vi "airplain.vi"(1 "steering":T1={"control"={"rudder"=-6, "aileron"=-15}, "rotate"={"pitch"=-22, "roll"=-18, "yaw"=158}, "pos"={"x"=0, "y"=0, "z"=-57}} {"control"."rudder" scale=-30.0..30.0; "control"."aileron" scale=-30.0..30.0; "rotate"."pitch" scale=-180.0..180.0; "rotate"."roll" scale=-180.0..180.0; "rotate"."yaw" scale=-180.0..180.0; "pos"."x" scale=-10.0..10.0; "pos"."y" scale=-20.0..20.0; "pos"."z" scale=-200.0..200.0}, 2 "center":cluster{"x":u32, "y":u32}={"x"=65, "y"=58}) -> (0 "picture out 2":picture)   [LabVIEW 2011]
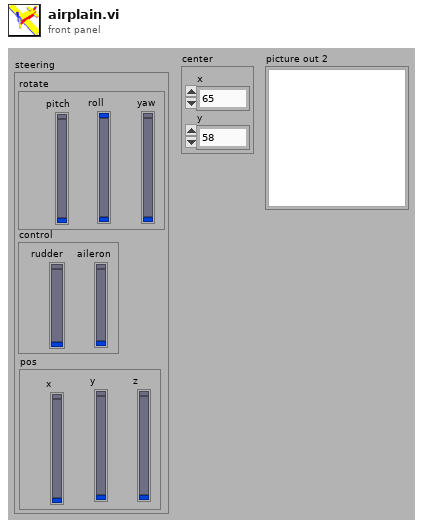
[diagram p1: front panel]
types:
  T1 = cluster{"control":cluster{"rudder":i32, "aileron":i32}, "rotate":cluster{"pitch":i32, "roll":i32, "yaw":i32}, "pos":cluster{"x":i32, "y":i32, "z":i32}}
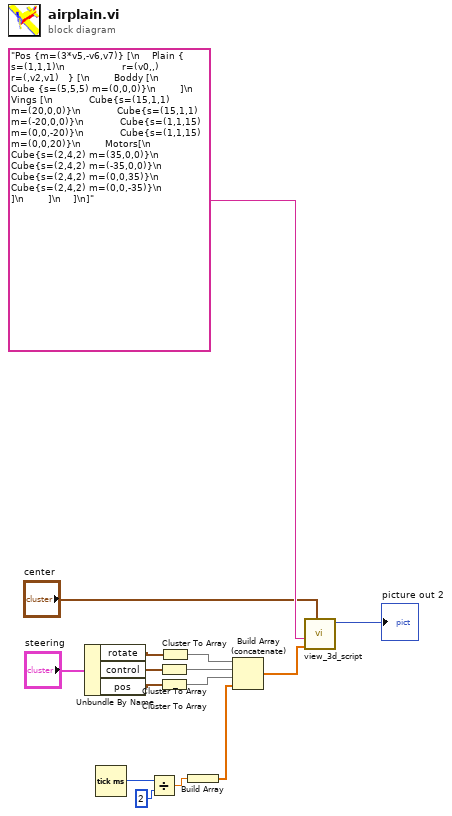
[diagram p0: block diagram]
diagram:
  n1 = Unbundle By Name("steering") -> ("rotate"=w1:cluster{"pitch":i32, "roll":i32, "yaw":i32}, "control"=w2:cluster{"rudder":i32, "aileron":i32}, "pos"=w3:cluster{"x":i32, "y":i32, "z":i32})
  n2 = Tick Count (ms)() -> (millisecond timer value=w10:u32)
  n3 = Divide(x=w10, y=u16 2) -> (x/y=w9:dbl)
  n4 = Cluster To Array(cluster=w2) -> (array=w14:i32[])
  n5 = Cluster To Array(cluster=w3) -> (array=w13:i32[])
  n6 = Cluster To Array(cluster=w1) -> (array=w15:i32[])
  n7 = Build Array(w9) -> (w12:dbl[])
  n8 = Build Array (concatenate)(w15, w14, w13, w12) -> (w8:dbl[])
  n9 = call "view_3d_script.vi"("center"="center", "variables"=w8, "script"="Pos {m=(3*v5,-v6,v7)} [\n    Plain { s=(1,1,1)\n                   r=(v0,,)  r=(,v2,v1)   } [\n        Boddy [\n            Cube {s=(5,5,5) m=(0,0,0)}\n        ]\n        Vings [\n            Cube{s=(15,1,1) m=(20,0,0)}\n            Cube{s=(15,1,1)  m=(-20,0,0)}\n            Cube{s=(1,1,15) m=(0,0,-20)}\n            Cube{s=(1,1,15)  m=(0,0,20)}\n        Motors[\n                Cube{s=(2,4,2) m=(35,0,0)}\n                Cube{s=(2,4,2) m=(-35,0,0)}\n                Cube{s=(2,4,2) m=(0,0,35)}\n                Cube{s=(2,4,2) m=(0,0,-35)}\n                    ]\n        ]\n    ]\n]") -> ("picture out"=→"picture out 2":picture)  [unwired: 3 in, 2 out]
